vi "Toggle Component Display.vi"(8 "error in":errorcluster, 9 "Show":bool, 10 "Identifier":string, 11 "Base Software in":refnum<class "Base Software.lvclass">) -> (0 "error out":errorcluster, 3 "Base Software out":refnum<class "Base Software.lvclass">)   [LabVIEW 2019, in "Base Software.lvlib" / "Main.lvlib" / "Base Software.lvclass"]
uses:
  Project/Base Software.lvclass
  Project/Base Software.lvclass/Base Software.ctl
  builds/Engine/Panel Manager.lvlibp/Panel Actor Messages/Show Panel Msg/Show Panel Msg.lvclass
  builds/Engine/Panel Manager.lvlibp/Panel Actor Messages/Hide Panel Msg/Hide Panel Msg.lvclass
  builds/Engine/Engine.lvlibp/Engine Messages/Adjust Splitter Msg/Adjust Splitter Msg.lvclass
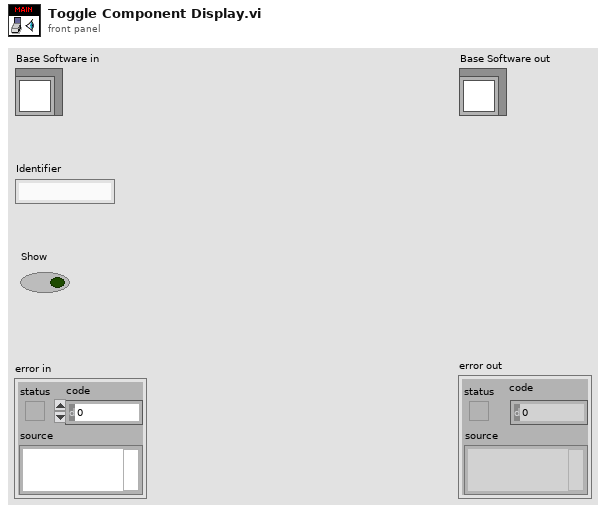
[diagram p1: front panel]
types:
  T1 = typedef "Base Software.lvlib/Main.lvlib/Base Software.lvclass/Panel_Positions.ctl" = enum16{"Prime", "Right", "Bottom", "Left", "Mission"}
  T2 = typedef "Base Software.lvlib/Main.lvlib/Base Software.lvclass/Splitters.ctl" = cluster{"Splitter":refnum<vi>, "Initial":i32}
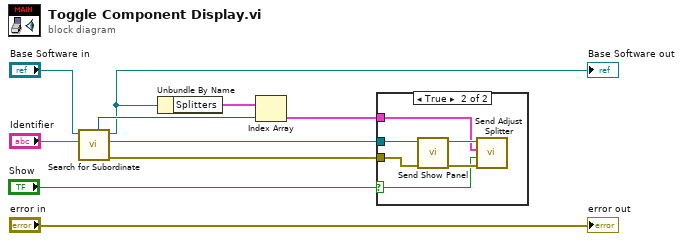
[diagram p0: block diagram]
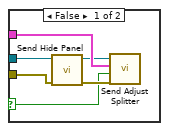
[diagram p2: hidden frame]
diagram:
  n1 = call "Search for Subordinate.vi"("Identifier"="Identifier", "Base Software in"="Base Software in") -> ("error out"=w6:errorcluster, "Enqueuer"=w7:refnum<class "Message Enqueuer.lvclass">, "Base Software out"=w1:refnum<class "Base Software.lvclass">, "Position"=w2:T1)  [unwired: 4 in, 2 out]
  "Base Software out" <- w1
  n2 = Unbundle By Name(w1) -> ("Splitters"=w4:T2[])
  n3 = Index Array(array=w4, index=w2) -> (element=w3:T2)
  n4 = case shown="True" "Show" {
    selector: "Show" -> [w11 w17]
    tunnel: w7 -> [w16 w22]
    tunnel: w6 -> [w15 w19]
    tunnel: w3 -> [w14 w18]
    frame False {
      n5 = call "Send Hide Panel.vi"("error in (no error)"=w15, "Message Enqueuer in"=w16) -> ("error out"=w13:errorcluster, "Message Enqueuer out"=w12:refnum<class "Message Enqueuer.lvclass">)  [unwired: 8 in]
      n6 = call "Send Adjust Splitter.vi"("error in (no error)"=w13, "Show"=w11, "Splitter Info"=w14, "Message Enqueuer"=w12) -> ()  [unwired: 6 in, 2 out]
    }
    frame True {
      n7 = call "Send Show Panel.vi"("Error In"=w19, "Message Enqueuer in"=w22) -> ("Error Out"=w21:errorcluster, "Message Enqueuer out"=w20:refnum<class "Message Enqueuer.lvclass">)  [unwired: 8 in]
      n8 = call "Send Adjust Splitter.vi"("error in (no error)"=w21, "Show"=w17, "Splitter Info"=w18, "Message Enqueuer"=w20) -> ()  [unwired: 6 in, 2 out]
    }
  }
  "error out" <- "error in"
